vi "array_intersperse.vi"(6 "position":enum16{"first", "last"}(ring), 8 "error in":errorcluster, 9 "every":i32=1 min=2, 10 "inject value":dbl format="%#_6p", 11 "input_values":dbl[](array[numeric])=[1000.0, 1090.0, 1180.0, 1270.0, 1360.0, 1450.0, 1540.0, 1630.0, 1720.0, 1810.0, 1900.0, 1990.0, 2080.0, 2170.0, 2260.0, 2350.0, 2440.0, 2530.0, 2620.0, 2710.0, 2800.0, 2890.0, 2980.0, 3070.0, 3160.0, 3250.0, 3340.0, 3430.0, 3520.0, 3610.0, 3700.0, 3790.0, 3880.0, 3970.0, 4060.0, 4150.0, 4240.0, 4330.0, 4420.0, 4510.0, 4600.0, 4690.0, 4780.0, 4870.0, 4960.0, 5050.0, 5140.0, 5230.0, 5320.0, 5410.0, 5500.0, 5590.0, 5680.0, 5770.0, 5860.0, 5950.0, 6040.0, 6130.0, 6220.0, 6310.0, 6400.0, 6490.0, 6580.0, 6670.0, 6760.0, 6850.0, 6940.0, 7030.0, 7120.0, 7210.0, 7300.0, 7390.0, 7480.0, 7570.0, 7660.0, 7750.0, 7840.0, 7930.0, 8020.0, 8110.0, 8200.0, 8290.0, 8380.0, 8470.0, 8560.0, 8650.0, 8740.0, 8830.0, 8920.0, 9010.0, 9100.0, 9190.0, 9280.0, 9370.0, 9460.0, 9550.0, 9640.0, 9730.0, 9820.0, 9910.0, 10000.0] format="%#_6p") -> (0 "error out":errorcluster, 1 "new_size":i32, 2 "initial_size":i32, 3 "result":dbl[](array[numeric])=[1000.0, 1090.0, 1180.0, 1270.0, 1360.0, 1450.0, 1540.0, 1630.0, 1720.0, 1810.0, 1900.0, 1990.0, 2080.0, 2170.0, 2260.0, 2350.0, 2440.0, 2530.0, 2620.0, 2710.0, 2800.0, 2890.0, 2980.0, 3070.0, 3160.0, 3250.0, 3340.0, 3430.0, 3520.0, 3610.0, 3700.0, 3790.0, 3880.0, 3970.0, 4060.0, 4150.0, 4240.0, 4330.0, 4420.0, 4510.0, 4600.0, 4690.0, 4780.0, 4870.0, 4960.0, 5050.0, 5140.0, 5230.0, 5320.0, 5410.0, 5500.0, 5590.0, 5680.0, 5770.0, 5860.0, 5950.0, 6040.0, 6130.0, 6220.0, 6310.0, 6400.0, 6490.0, 6580.0, 6670.0, 6760.0, 6850.0, 6940.0, 7030.0, 7120.0, 7210.0, 7300.0, 7390.0, 7480.0, 7570.0, 7660.0, 7750.0, 7840.0, 7930.0, 8020.0, 8110.0, 8200.0, 8290.0, 8380.0, 8470.0, 8560.0, 8650.0, 8740.0, 8830.0, 8920.0, 9010.0, 9100.0, 9190.0, 9280.0, 9370.0, 9460.0, 9550.0, 9640.0, 9730.0, 9820.0, 9910.0, 10000.0] format="%#_6p")   [LabVIEW 2017, in "tools.lvlib"]
uses:
  tools.lvlib
panel:
  out "remaining":i32
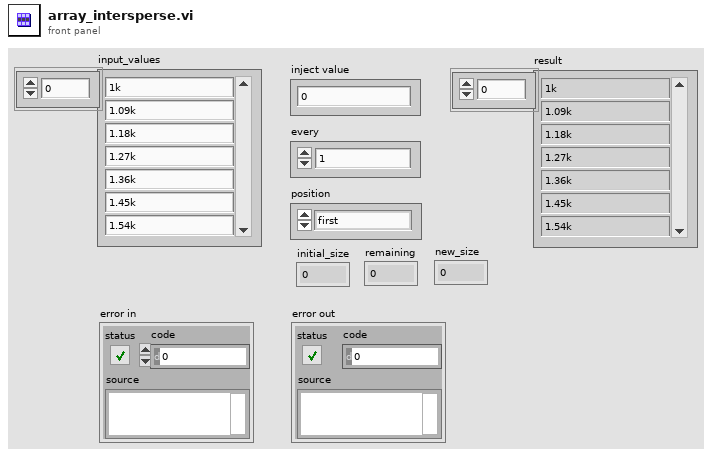
[diagram p1: front panel]
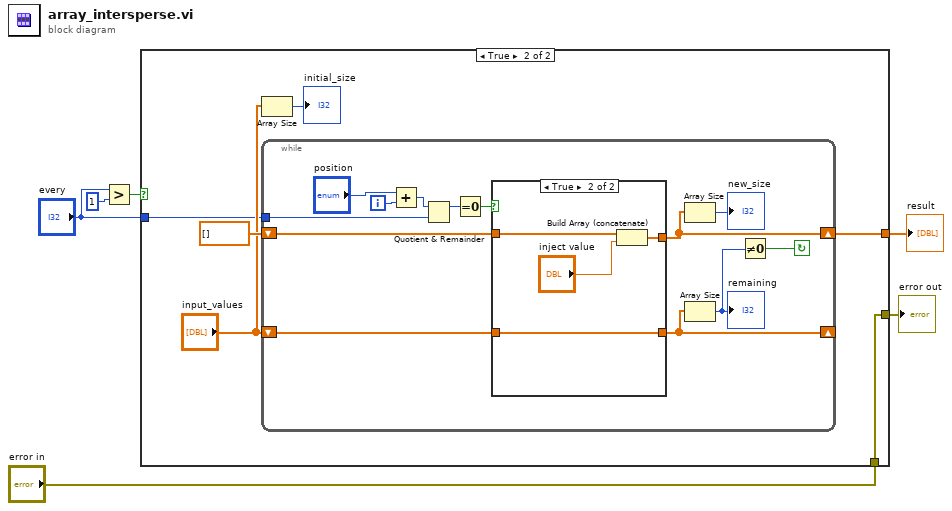
[diagram p0: block diagram]
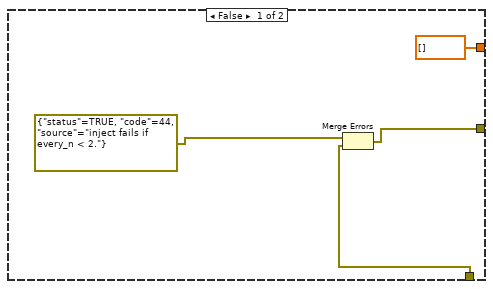
[diagram p2: hidden frame]
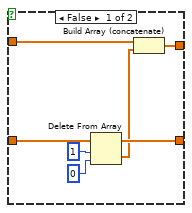
[diagram p3: hidden frame]
diagram:
  n1 = Greater?(x="every", y=1) -> (0:w5:bool)
  n2 = case shown="True" w5 {
    tunnel: [dbl[] [] ("input_values") w13] -> w4
    tunnel: "every" -> [_ w12]
    tunnel: [w7 w11] -> w2
    tunnel: "error in" -> [w8 w11]
    frame False {
      n3 = Merge Errors(errorcluster {"status"=TRUE, "code"=44, "source"="inject fails if every_n < 2."} ("error constant"), w8) -> (w7:errorcluster)
    }
    frame True {
      n4 = Array Size(array="input_values") -> (size(s)=→"initial_size":i32)
      n5 = while {
        shift-right: [w25] -> _
        shift-left: "input_values" -> [w26]
        shift-right: [w21] -> w13
        shift-left: dbl[] [] ("input_values") -> [w27]
        tunnel: w12 -> [w18]
        i -> [w19]
        stop <- w23 continue-if-true
        n6 = Add(x="position", y=w19) -> (x+y=w17:i32)
        n7 = Quotient & Remainder(x=w17, y=w18) -> (x-y*floor(x/y)=w29:i32)  [unwired: 1 out]
        n8 = Equal To 0?(x=w29) -> (x = 0?=w28:bool)
        n9 = case shown="True" w28 {
          tunnel: w27 -> [w32 w40]
          tunnel: [w33 w39] -> w21
          tunnel: w26 -> [w36 w37]
          tunnel: [w35 w37] -> w25
          frame False {
            n10 = Delete From Array(array=w36, length=1, index=0) -> (deleted portion=w34:dbl[], array with subset deleted=w35:dbl[])
            n11 = Build Array (concatenate)(w32, w34) -> (w33:dbl[])
          }
          frame True {
            n12 = Build Array (concatenate)(w40, "inject value") -> (w39:dbl[])
          }
        }
        n13 = Array Size(array=w21) -> (size(s)=→"new_size":i32)
        n14 = Array Size(array=w25) -> (size(s)=w24:i32)
        "remaining" <- w24
        n15 = Not Equal To 0?(x=w24) -> (x != 0?=w23:bool)
      }
    }
  }
  "result" <- w4
  "error out" <- w2
